vi "8.vi"() -> ()   [LabVIEW 2017]
panel:
  out "时间/s":dbl
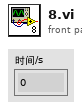
[diagram p1: front panel]
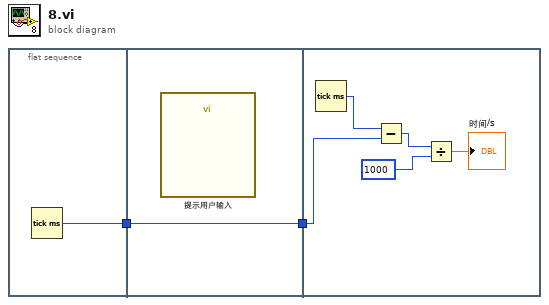
[diagram p0: block diagram]
diagram:
  n1 = flat-sequence {
    tunnel: [w3] -> w2
    tunnel: w2 -> [w4]
    tunnel: [w4] -> w1
    tunnel: w1 -> [w8]
    frame #0 {
      n2 = Tick Count (ms)() -> (millisecond timer value=w3:u32)
    }
    frame #1 {
      n3 = call "提示用户输入"() -> ()  [unwired: 17 in, 3 out]
    }
    frame #2 {
      n4 = Tick Count (ms)() -> (millisecond timer value=w9:u32)
      n5 = Subtract(x=w9, y=w8) -> (x-y=w7:u32)
      n6 = Divide(x=w7, y=u32 1000) -> (x/y=→"时间/s":dbl)
    }
  }
